vi "Periodic Tasks.vi"(8 "error in":errorcluster) -> ()   [LabVIEW 2015]
doc: "This VI runs in parallel to other tasks. It can contain as many user-defined periodic loops as you need. These can carry out PID or other sorts of timed response."
uses:
  <vilib>/Rock Robotics/WPI/Relay/WPI_RelayValue.ctl
  <vilib>/Rock Robotics/SystemInterfaces/spilib/spi_bus.ctl
  <vilib>/addons/control/pid/pid.llb/PID Structure.ctl
  <vilib>/Rock Robotics/WPI/CAN/TalonSRX/WPI_CANTalonSRX_APIControlMode.ctl
  <vilib>/Rock Robotics/Network Tables/NT Read Number.vi
  Robot Global Data.vi
  <vilib>/Rock Robotics/Network Tables/NT Write Number.vi
  <vilib>/Rock Robotics/WPI/Solenoid/Deprecated/WPI_SolenoidSetBool.vi
  VIs/ConvertVoltageToPercentVbs.vi
  <vilib>/Rock Robotics/Network Tables/NT Write Boolean.vi
  <vilib>/addons/control/pid/pid.llb/PID Control Input Filter (DBL).vi
  <vilib>/addons/control/pid/pid.llb/PID Structure Conversion (DBL).vi
  <vilib>/addons/control/pid/pid.llb/PID (DBL).vi
  <vilib>/Rock Robotics/Network Tables/NT Read Boolean.vi
  <vilib>/Rock Robotics/WPI/Gyro/WPI_GyroXRS450_SPI_Open.vi
  <vilib>/addons/control/pid/NI_PID_pid.lvlib
panel:
  out "Arm Motor Output":dbl
  out "Normalized Value":dbl
  out "Arm Angle":dbl
  in  "Current Limit 2":dbl=5.0
  in  "Driving Power 2":dbl=0.4
  out "current (A)":dbl
  in  "PID Arm Good Range":dbl=3.0
  out "Arm Angle PID 3":dbl
  in  "Arm Angle PID 2":T1={"proportional gain (Kc)"=0.018, "integral time (Ti, min)"=1.25, "derivative time (Td, min)"=1e-05}
  out "Arm PID Output Graph":dbl(graph)
  out "Arm PID Output":dbl
  out "Arm Setpoint PID":dbl
  in  "Arm PID Output Range":cluster{"output high":dbl, "output low":dbl}={"output high"=0.5, "output low"=-0.5} {"output low" format="%.2f"; "output high" format="%.2f"}
  in  "Holding Power":dbl=0.1
  in  "Driving Power":dbl=0.6
  in  "Current Limit":dbl=8.0
  out "Scaled Vision x":dbl
  out "Ball Holder Voltage":dbl
  out "Gyro Resetting":bool
  out "SHOOT":bool
  out "Ball Holder":bool
  in  "D Left":dbl
  in  "D Right":dbl
  out "R Error":dbl(graph)
  out "L Error":dbl(graph)
  in  "I Right":dbl
  in  "I Left":dbl
  out "Shooter Data":T2={"Arm Angle"={"D4"=44.0, "Fender"=69.0, "Low Goal"=-1.0, "Bottom"=-3.0}, "Wheel Speed"={"D4"=4500.0, "Fender"=3600.0, "Low Goal"=3000.0, "Intake"=-11.0}}
  in  "Wheel Speed Setpoints":T3={"D4"=3450.0, "Fender"=3500.0, "Low Goal"=2500.0, "Intake"=-13.0}
  in  "Arm Angle Setpoints":T4={"D4"=38.0, "Fender"=72.0, "Low Goal"=-1.0, "Bottom"=0.0}
  out "Angle":dbl
  in  "Reset Gyro":bool
  out "Speed Closed Loop Plots R":cluster{dbl, "Sensor Velocity":dbl}(graph)
  out "SensorRPM Velocity RPM R":dbl
  out "Target RPM R":dbl
  out "Target RPM L":dbl
  out "SensorRPM Velocity RPM L":dbl
  out "Speed Closed Loop Plots L":cluster{dbl, "Sensor Velocity":dbl}(graph)
  in  "P Right":dbl=0.1
  in  "F Right":dbl=0.02417
  in  "P Left":dbl=0.11
  in  "F Left":dbl=0.025837
  out "Vision X Dashboard":dbl
  out "Vision Y Dashboard":dbl
  out "Average Distance":dbl
  # "Sensor Stuff"
  # "Random Stuff"
  # "Vision Stuff"
  # "Shooter Data"
  # "Arm Angle Control"
  # "-3"
  # "OLD F\n3300"
  # "Shooter Wheel Control"
  # "RIGHT"
  # "50\n50"
  # "Delays to compensate for wheel speed.\n\n1: Wait for wheels to spin up before piston fires\n2: Keep wheels spun up after piston fires"
  # "LEFT"
  # ".45\n.37\n\n.15\n.025"
  # "Arm Angle"
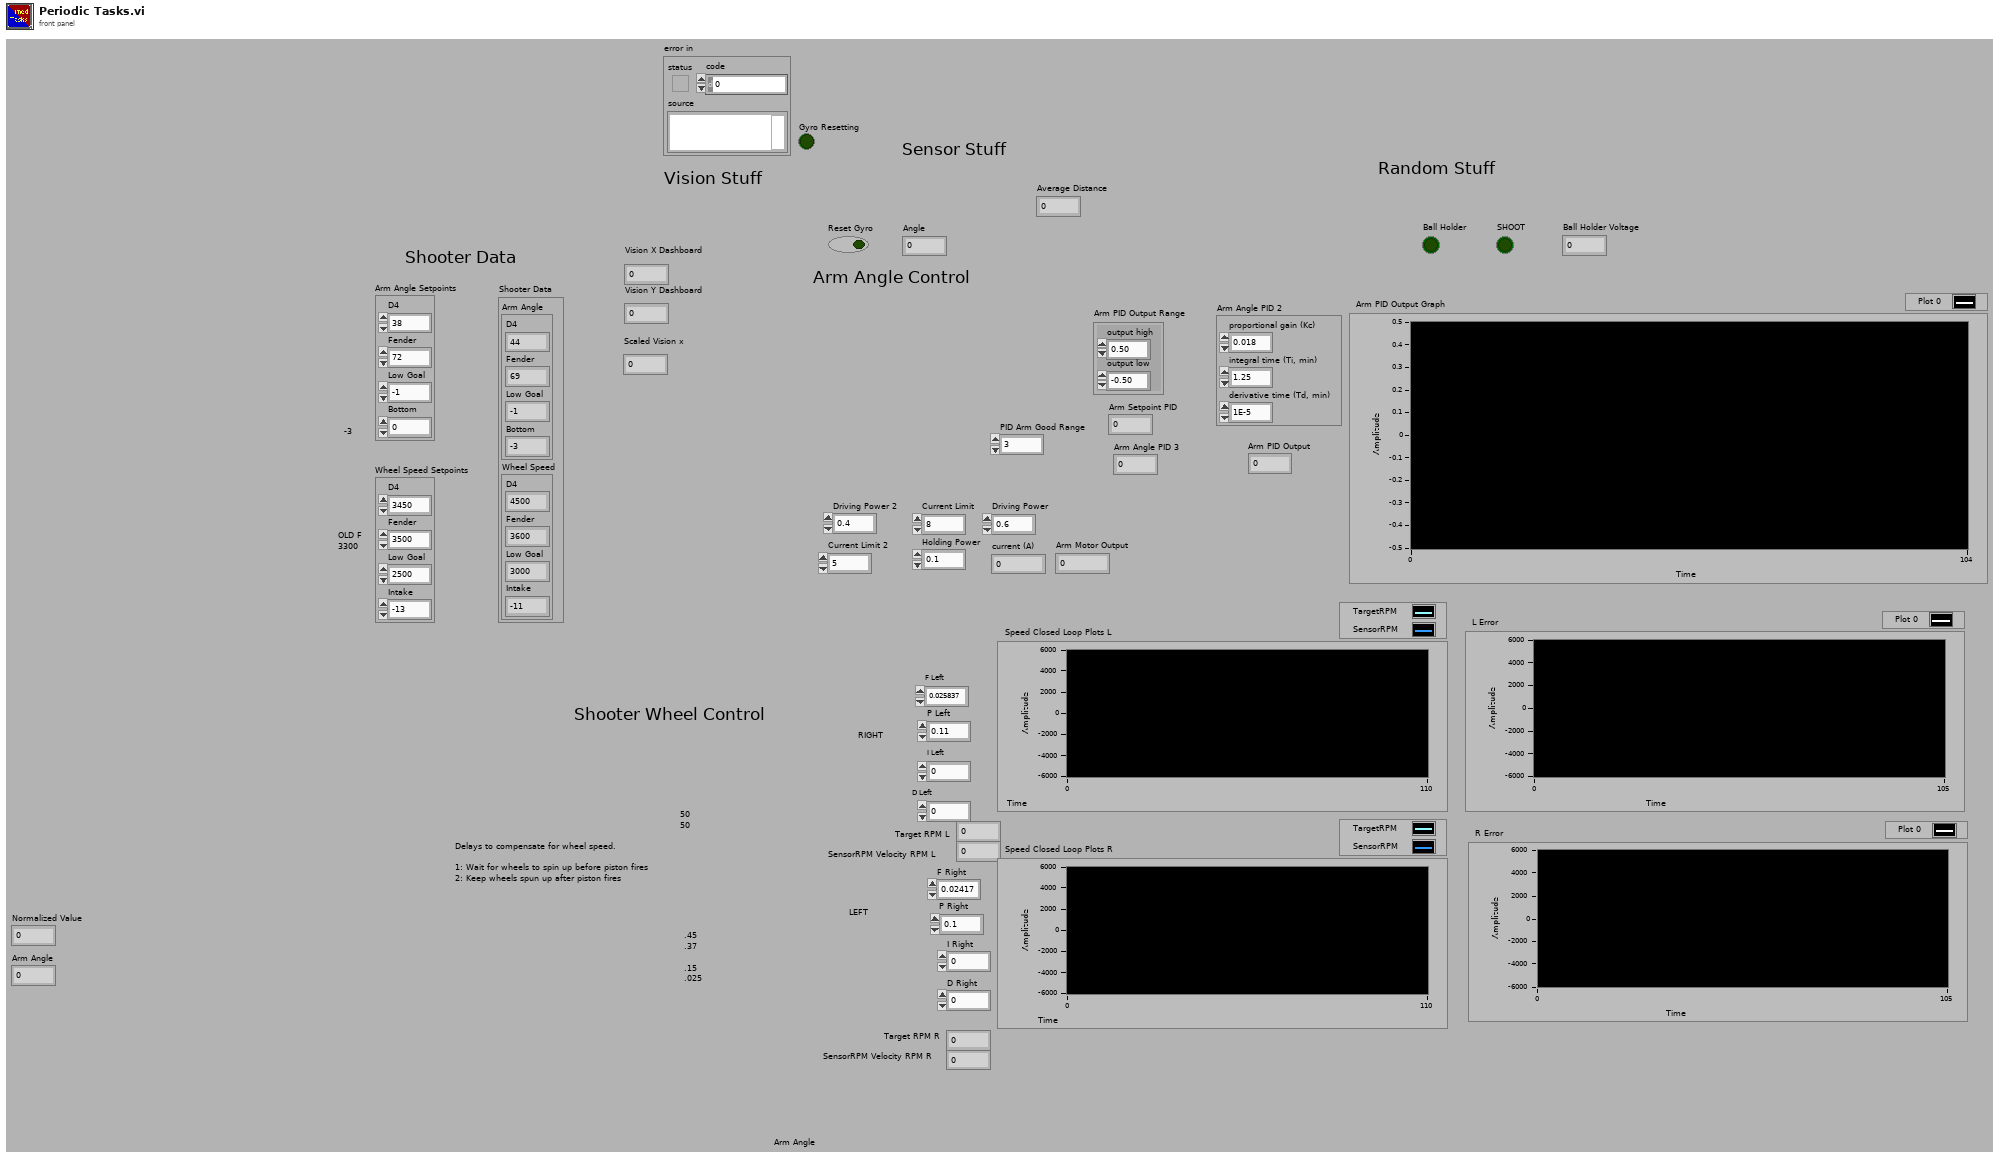
[diagram p1: front panel]
types:
  T1 = cluster{"proportional gain (Kc)":dbl, "integral time (Ti, min)":dbl, "derivative time (Td, min)":dbl}
  T2 = cluster{"Arm Angle":cluster{"D4":dbl, "Fender":dbl, "Low Goal":dbl, "Bottom":dbl}, "Wheel Speed":cluster{"D4":dbl, "Fender":dbl, "Low Goal":dbl, "Intake":dbl}}
  T3 = cluster{"D4":dbl, "Fender":dbl, "Low Goal":dbl, "Intake":dbl}
  T4 = cluster{"D4":dbl, "Fender":dbl, "Low Goal":dbl, "Bottom":dbl}
  T5 = typedef "WPI_PotentiometerDevRef.ctl" = cluster{"DevStatus":errorcluster, "Analog Channel":T6, "Invert Output":bool}
  T6 = typedef "FPGA_AIChannel.ctl" = enum8{"AI 0", "AI 1", "AI 2", "AI 3", "AI MXP 0", "AI MXP 1", "AI MXP 2", "AI MXP 3", "Invalid"}
  T7 = typedef "NI_PID_pid.lvlib/PID Structure.ctl" = u16
  T8 = typedef "WPI_MotorControlDeviceRef.ctl" = cluster{"DeviceStatus":errorcluster, "Type":T9, "PWM":cluster{"PWM Channel":T10, "DeadBand":T11}, "CAN":cluster{"Device Number":u8, "Control Mode":T12, "Semaphore":T13, "Max Vout":dbl, "TalonSRX Control Mode":T14}, "Invert":bool}
  T9 = typedef "WPI_MotorControlType.ctl" = enum16{"PWM", "CAN", "CANTalonSRX"}
  T10 = typedef "FPGA_DIOPWMChannel.ctl" = enum8{"PWM 0", "PWM 1", "PWM 2", "PWM 3", "PWM 4", "PWM 5", "PWM 6", "PWM 7", "PWM 8", "PWM 9", "PWM MXP 0", "PWM MXP 1", "PWM MXP 2", "PWM MXP 3", "PWM MXP 4", "PWM MXP 5", "PWM MXP 6", "PWM MXP 7", "PWM MXP 8", "PWM MXP 9", "Invalid"}
  T11 = typedef "WPI_PWMDeadband.ctl" = cluster{"Name":string, "maxPositivePwm":i32, "minPositivePwm":i32, "centerPwm":i32, "maxNegativePwm":i32, "minNegativePwm":i32, "angularRange":u16}
  T12 = typedef "WPI_CANJaguar_ControlMode.ctl" = enum8{"Percent VBus", "Current", "Speed", "Position", "Voltage"}
  T13 = typedef "Semaphore RefNum" = refnum<k1>
  T14 = typedef "WPI_CANTalonSRX_APIControlMode.ctl" = enum8{"Percent VBus", "Speed", "Position", "Slave", "Unchanged / Invalid", "Voltage Compensation", "Current", "Motion Profile"}
  T15 = typedef "WPI_EncoderDevRef.ctl" = cluster{"DevStatus":errorcluster, "EncoderIndex":T16, "CounterIndex":T17, "DistancePerCount":dbl, "Decoding Type":T18}
  T16 = typedef "FPGA_EncoderIdx.ctl" = enum8{"Enc 0", "Enc 1", "Enc 2", "Enc 3", "Enc 4", "Enc 5", "Enc 6", "Enc 7", "Invalid"}
  T17 = typedef "FPGA_CounterCtrSystemIndex.ctl" = enum8{"Ctr 0", "Ctr 1", "Ctr 2", "Ctr 3", "Ctr 4", "Ctr 5", "Ctr 6", "Ctr 7", "Invalid"}
  T18 = typedef "WPI_EncoderType.ctl" = enum16{"1x", "2x", "4x"}
  T19 = typedef "WPI_GyroDevRef.ctl" = cluster{"DevStatus":errorcluster, "Analog Channel":T6, "Offset":dbl, "Gain (VoltsPerDegree/Second)":dbl, "Gyro Type":enum16{"Analog", "XRS450"}, "Handle":i32, "SPI Bus":T20, "Device Found":bool, "Sample Rate":dbl, "Calibrate On Open":bool}
  T20 = typedef "spi_bus.ctl" = enum16{"SPI On-Board, CS0", "SPI On-Board, CS1", "SPI On-Board, CS2", "SPI On-Board, CS3", "SPI MXP", "Invalid"}
  T21 = typedef "WPI_RelayValue.ctl" = enum16{"Off", "On", "Forward", "Reverse"}
  T22 = typedef "WPI_SolenoidDevRef.ctl" = cluster{"DevStatus":errorcluster, "Pneumatics Control Module":u8, "Forward Solenoid Channel":T23, "Reverse Solenoid Channel":T23}
  T23 = typedef "WPI_SolenoidChannel.ctl" = enum8{"Solenoid 0", "Solenoid 1", "Solenoid 2", "Solenoid 3", "Solenoid 4", "Solenoid 5", "Solenoid 6", "Solenoid 7", "Invalid"}
  T24 = typedef "WPI_RelayDevRef.ctl" = cluster{"DevStatus":errorcluster, "Relay Channel":T25, "Relay Direction":T26}
  T25 = typedef "FPGA_DIORelayChannel.ctl" = enum8{"Relay 0", "Relay 1", "Relay 2", "Relay 3", "Invalid"}
  T26 = typedef "WPI_RelayDirection.ctl" = enum16{"Both directions", "Forward only", "Reverse only"}
  T27 = typedef "WPI_CANTalonSRX_GlobalStatus.ctl" = cluster{"Applied Throttle":dbl, "Module Enabled":bool, "CAN Error":errorcluster, "Closed Loop Error":dbl, "Forward Limit Switch Closed":bool, "Reverse Limit Switch Closed":bool, "Sensor Position":dbl, "Sensor Velocity":dbl, "Current":dbl, "Sticky Fault - Over Temp":bool, "Sticky Fault - Under Voltage":bool, "Sticky Fault - Forward Limit":bool, "Sticky Fault - Reverse Limit":bool, "Sticky Fault - Forward Soft Limit":bool, "Sticky Fault - Reverse Soft Limit":bool, "Brake is Enabled":bool, "Encoder Position":dbl, "Encoder Velocity":dbl, "Encoder Index Count":dbl, "Encoder A Pin State":bool, "Encoder B Pin State":bool, "Encoder Index Pin State":bool, "Analog In":dbl, "Analog In Velocity":dbl, "Temperature (C)":dbl, "Battery Voltage":dbl, "Control 5 Is Supported":bool, "Current Profile Slot Select":dbl, "Pos Div 8":bool, "Vel Div 4":bool, "Pulse Width Position":i32, "Pulse Width Velocity":i32, "Pulse Width Rise To Rise (us)":i32, "Pulse Width Rise To Fall (us)":i32, "Mot Prof Active Is Under Run":bool, "Mot Prof Active Has Under Run":bool, "Mot Prof Active Is Last":bool, "Mot Prof Active Velocity Only":bool, "Mot Prof Active Is Valid":bool, "Mot Prof Buffer Is Full":bool, "Mot Prof Active Profile Slot Select":i32, "Mot Prof NextID":i32, "Mot Prof Count":i32, "Mot Prof Active Velocity":dbl, "Mot Prof Active Position":dbl, "Mot Prof Output Enable":i32}
  T28 = cluster{"Shooter Setpoint Speed (RPM)":dbl, "Sensor Velocity":dbl}
  T29 = typedef "WPI_AnalogChannelDevRef.ctl" = cluster{"DevStatus":errorcluster, "Analog Channel":T6}
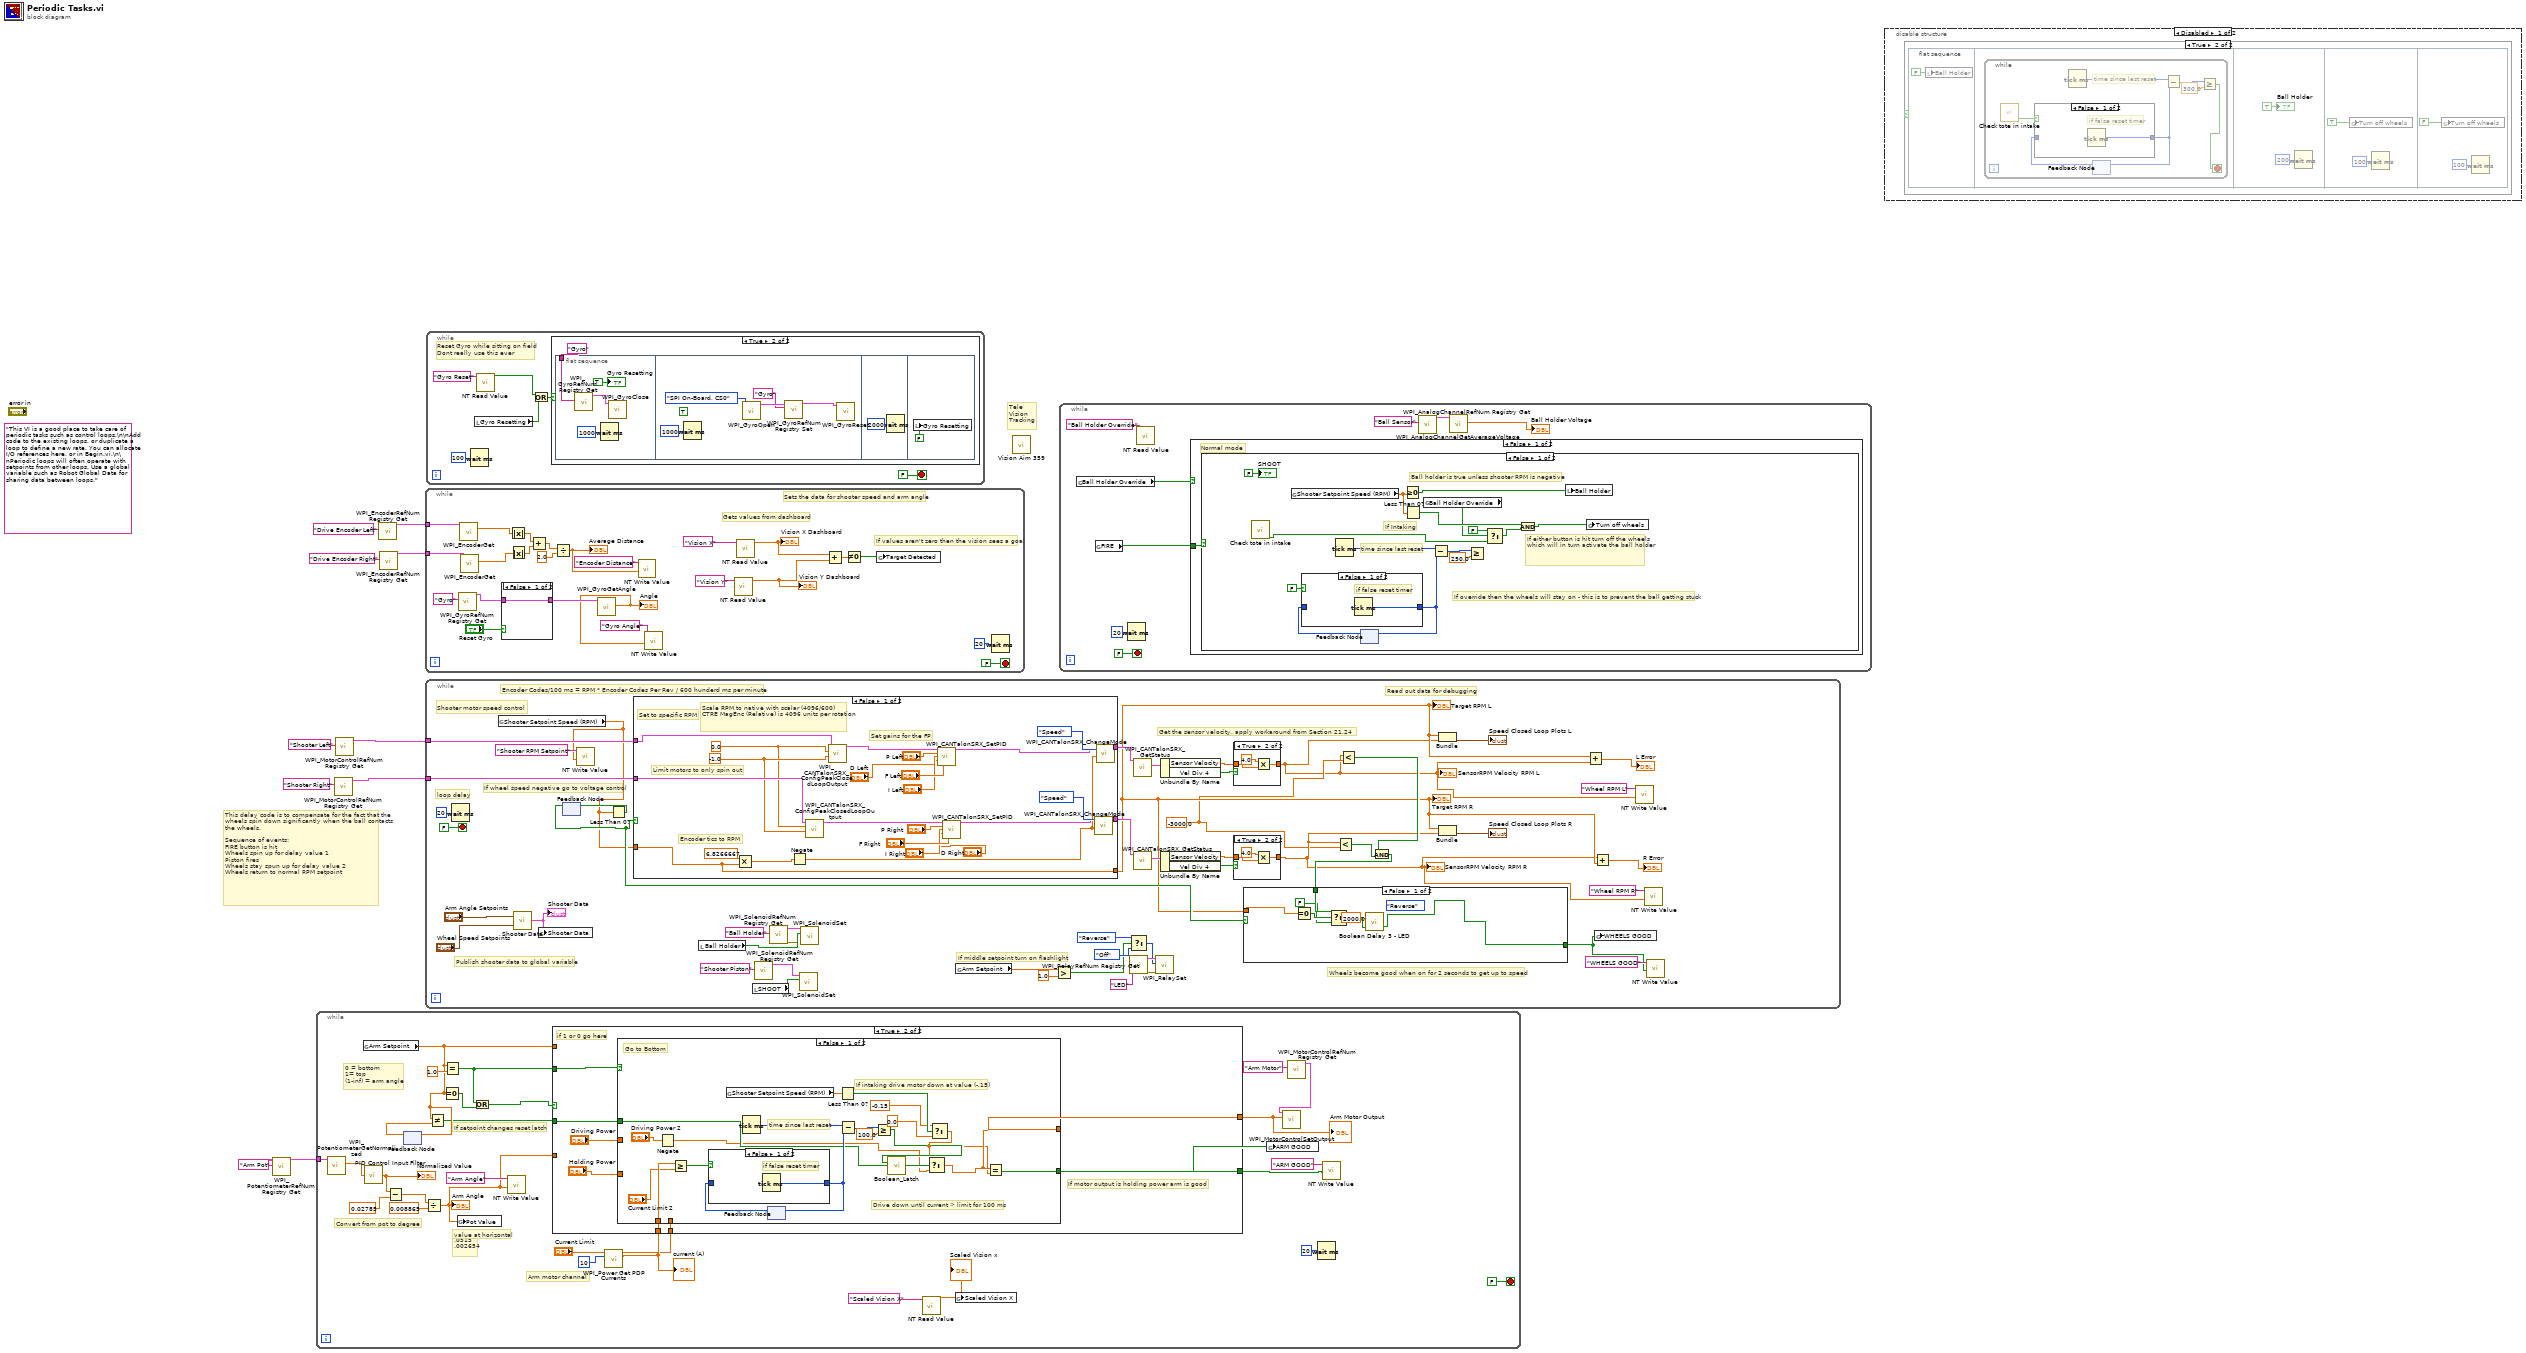
[diagram p0: block diagram]
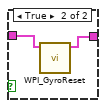
[diagram p2: hidden frame]
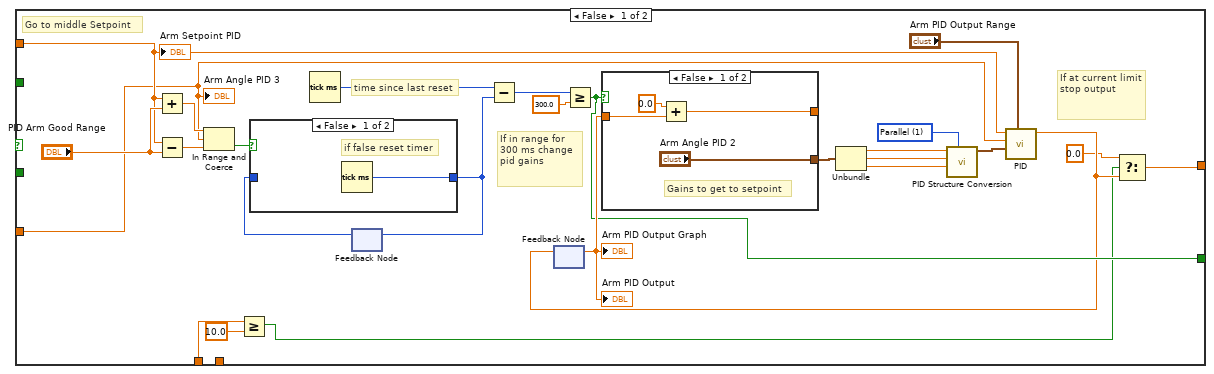
[diagram p6: hidden frame]
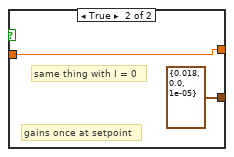
[diagram p8: hidden frame]
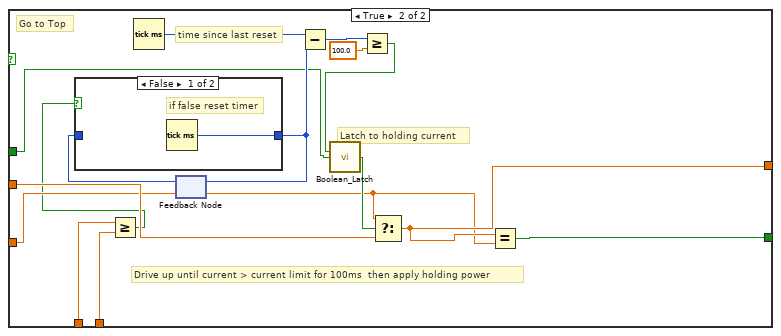
[diagram p10: hidden frame]
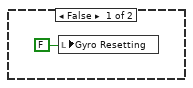
[diagram p12: hidden frame]
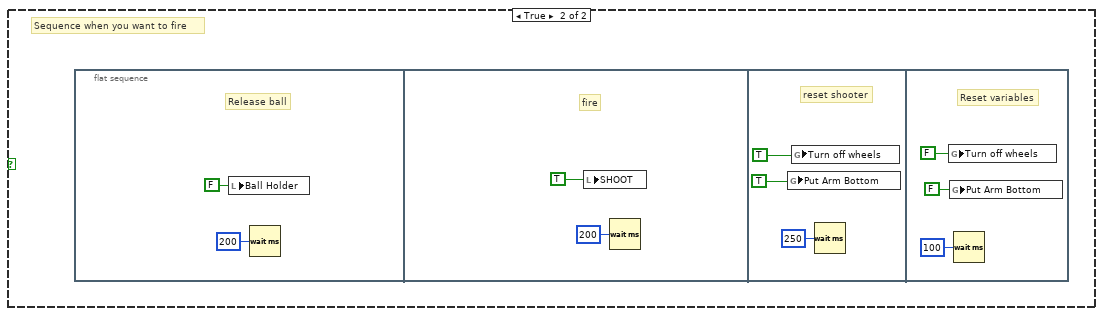
[diagram p14: hidden frame]
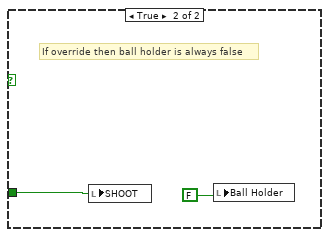
[diagram p15: hidden frame]
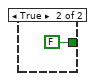
[diagram p16: hidden frame]
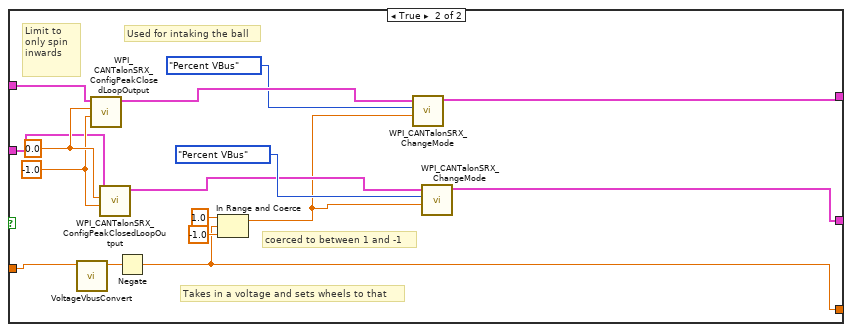
[diagram p19: hidden frame]
diagram:
  (unwired) "This VI is a good place to take care of periodic tasks such as control loops.\n\nAdd code to the existing loops, or duplicate a loop to define a new rate. You can allocate I/O references here, or in Begin.vi.\n\nPeriodic loops will often operate with setpoints from other loops. Use a global variable such as Robot Global Data for sharing data between loops."
  # "Tele \nVision\nTracking"
  # "This delay code is to compensate for the fact that the wheels spin down significantly when the ball contacts the wheels.\n\nSequence of events:\nFIRE button is hit\nWheels spin up for delay value 1\nPiston fires\nWheels stay spun up for delay value 2\nWheels return to normal RPM setpoint"
  n1 = call <vilib>:"WPI_PotentiometerRefNum Registry Get.vi"("refnum name"="Arm Pot") -> ("PotDevRef"=w1:T5)  [unwired: 9 in, 1 out]
  n2 = while {
    tunnel: w1 -> [w17]
    stop <- FALSE stop-if-true
    # "If setpoint changes reset latch"
    # "0 = bottom\n1= top \n(1-inf) = arm angle"
    # "Convert from pot to degree"
    # "value at horizontal"
    # "old\n.0515\n.002654"
    # "Arm motor channel"
    n3 = call <vilib>:"WPI_PotentiometerGetNormalized.vi"("PotDevRef"=w17) -> ("Normalized Value"=w20:dbl)  [unwired: 8 in, 2 out]
    n4 = global read "Robot Global Data.vi" "Arm Setpoint"() -> (w13:dbl)
    n5 = call-poly <vilib>:"PID Control Input Filter.vi"("input"=w20) -> ("output"=w19:dbl)  [unwired: 4 in]
    "Normalized Value" <- w19
    n6 = Subtract(x=w19, y=0.02785) -> (x-y=w23:dbl)
    n7 = feedback-in #1(w13) -> ()
    n8 = feedback #1() -> (w25:dbl)  [unwired: 1 in]
    n9 = Divide(x=w23, y=0.008865) -> (x/y=w18:dbl)
    "Arm Angle" <- w18
    n10 = Not Equal?(x=w13, y=w25) -> (x != y?=w12:bool)
    n11 = Equal To 0?(x=w13) -> (x = 0?=w36:bool)
    n12 = Equal?(x=w13, y=1.0) -> (x = y?=w35:bool)
    n13 = global write "Robot Global Data.vi" "Pot Value"(w18) -> ()
    n14 = Or(x=w35, y=w36) -> (x .or. y?=w11:bool)
    n15 = call-poly <vilib>:"NT Write Value.vi"("Numeric"=w18, "Name"="Arm Angle") -> ()  [unwired: 9 in, 1 out]
    n16 = call <vilib>:"WPI_Power Get PDP Currents.vi"("PDP Channel"=10) -> ("current (A)"=w33:dbl)  [unwired: 12 in, 2 out]
    "current (A)" <- w33
    n17 = case shown="True" w11 {
      tunnel: w35 -> [_ w79]
      tunnel: w33 -> [w43 w78]
      tunnel: "Current Limit" -> [_ w77]
      tunnel: [w45 w74] -> w30
      tunnel: w13 -> [w46 _]
      tunnel: [w41 w73] -> w14
      tunnel: w12 -> [_ w72]
      tunnel: w18 -> [w44 _]
      frame False {
        w50 = T7 1 items=["Academic (Standard)", "Parallel", "Series"] ("PID structure")
        # "If in range for 300 ms change pid gains"
        # "If at current limit stop output"
        # "time since last reset"
        # "Go to middle Setpoint"
        n18 = Add(x=w46, y="PID Arm Good Range") -> (x+y=w48:dbl)
        n19 = Subtract(x=w46, y="PID Arm Good Range") -> (x-y=w49:dbl)
        n20 = In Range and Coerce(upper limit=w48, x=w44, lower limit=w49) -> (In Range?=w62:bool)  [unwired: 1 out]
        n21 = Greater Or Equal?(x=w43, y=10.0) -> (x >= y?=w38:bool)
        n22 = Tick Count (ms)() -> (millisecond timer value=w57:u32)
        n23 = feedback #2() -> (w60:u32)  [unwired: 1 in]
        n24 = case shown="False" w62 {
          tunnel: [w64 w65] -> w58
          tunnel: w60 -> [_ w65]
          frame False {
            # "if false reset timer"
            n25 = Tick Count (ms)() -> (millisecond timer value=w64:u32)
          }
          frame True {
            # "if true don't reset timer"
          }
        }
        n26 = feedback-in #2(w58) -> ()
        n27 = Subtract(x=w57, y=w58) -> (x-y=w59:u32)
        n28 = feedback #3() -> (w56:dbl)  [unwired: 1 in]
        "Arm PID Output" <- w56
        "Arm PID Output Graph" <- w56
        n29 = Greater Or Equal?(x=w59, y=300.0 ("Delay (ms)")) -> (x >= y?=w45:bool)
        n30 = case shown="False" w45 {
          tunnel: ["Arm Angle PID 2" T1 {"proportional gain (Kc)"=0.018, "integral time (Ti, min)"=0.0, "derivative time (Td, min)"=1e-05} ("cluster")] -> w47
          tunnel: [w66 w70] -> _
          tunnel: w56 -> [w68 w70]
          frame False {
            # "Gains to get to setpoint"
            n31 = Add(x=0.0, y=w68) -> (x+y=w66:dbl)
          }
          frame True {
            # "same thing with I = 0"
            # "gains once at setpoint"
          }
        }
        n32 = Unbundle(w47) -> ("proportional gain (Kc)"=w55:dbl, "integral time (Ti, min)"=w54:dbl, "derivative time (Td, min)"=w53:dbl)
        n33 = call-poly <vilib>:"PID Structure Conversion.vi"("PID structure"=w50, "derivative"=w53, "integral"=w54, "proportional"=w55) -> ("PID gains"=w52:T1)  [unwired: 7 in]
        n34 = call-poly <vilib>:"PID.vi"("output range"="Arm PID Output Range", "PID gains"=w52, "process variable"=w44, "setpoint"=w46) -> ("output"=w40:dbl)  [unwired: 6 in, 1 out]
        n35 = feedback-in #3(w40) -> ()
        n36 = Select(t=0.0, s=w38, f=w40) -> (s? t:f=w41:dbl)
        "Arm Setpoint PID" <- w46
        "Arm Angle PID 3" <- w44
      }
      frame True {
        # "If motor output is holding power arm is good"
        # "if 1 or 0 go here"
        n37 = case shown="False" w79 {
          tunnel: w78 -> [w99 w116]
          tunnel: w77 -> [_ w115]
          tunnel: "Holding Power" -> [_ w110]
          tunnel: "Driving Power" -> [_ w111]
          tunnel: [w98 w114] -> w74
          tunnel: [w96 w112] -> w73
          tunnel: w72 -> [w88 w102]
          frame False {
            # "If intaking drive motor down at value (-.15)"
            # "Drive down until current > limit for 100 ms"
            # "time since last reset"
            # "Go to Bottom"
            n38 = Negate(x="Driving Power 2") -> (-x=w87:dbl)
            n39 = Greater Or Equal?(x=w99, y="Current Limit 2") -> (x >= y?=w90:bool)
            n40 = global read "Robot Global Data.vi" "Shooter Setpoint Speed (RPM)"() -> (w82:dbl)
            n41 = Tick Count (ms)() -> (millisecond timer value=w95:u32)
            n42 = feedback #4() -> (w91:u32)  [unwired: 1 in]
            n43 = case shown="False" w90 {
              tunnel: [w100 w101] -> w94
              tunnel: w91 -> [_ w101]
              frame False {
                # "if false reset timer"
                n44 = Tick Count (ms)() -> (millisecond timer value=w100:u32)
              }
              frame True {
                # "if true don't reset timer"
              }
            }
            n45 = feedback-in #4(w94) -> ()
            n46 = Less Than 0?(x=w82) -> (x < 0?=w81:bool)
            n47 = Subtract(x=w95, y=w94) -> (x-y=w93:u32)
            n48 = Greater Or Equal?(x=w93, y=100.0 ("Delay (ms)")) -> (x >= y?=w89:bool)
            n49 = call "Boolean_Latch.vi"("Latch Control"=w89, "Reset"=w88) -> ("Latched?"=w97:bool)  [unwired: 13 in]
            n50 = Select(t=-0.15, s=w81, f=0.0) -> (s? t:f=w83:dbl)
            n51 = Select(t=w83, s=w97, f=w87) -> (s? t:f=w96:dbl)
            n52 = Equal?(x=w96, y=w83) -> (x = y?=w98:bool)
          }
          frame True {
            # "Latch to holding current"
            # "Drive up until current > current limit for 100ms  then apply holding power"
            # "time since last reset"
            # "Go to Top"
            n53 = Greater Or Equal?(x=w116, y=w115) -> (x >= y?=w103:bool)
            n54 = Tick Count (ms)() -> (millisecond timer value=w109:u32)
            n55 = feedback #5() -> (w105:u32)  [unwired: 1 in]
            n56 = case shown="False" w103 {
              tunnel: [w117 w118] -> w108
              tunnel: w105 -> [_ w118]
              frame False {
                # "if false reset timer"
                n57 = Tick Count (ms)() -> (millisecond timer value=w117:u32)
              }
              frame True {
                # "if true don't reset timer"
              }
            }
            n58 = feedback-in #5(w108) -> ()
            n59 = Subtract(x=w109, y=w108) -> (x-y=w107:u32)
            n60 = Greater Or Equal?(x=w107, y=100.0 ("Delay (ms)")) -> (x >= y?=w104:bool)
            n61 = call "Boolean_Latch.vi"("Latch Control"=w104, "Reset"=w102) -> ("Latched?"=w113:bool)  [unwired: 13 in]
            n62 = Select(t=w110, s=w113, f=w111) -> (s? t:f=w112:dbl)
            n63 = Equal?(x=w112, y=w110) -> (x = y?=w114:bool)
          }
        }
      }
    }
    "Arm Motor Output" <- w14
    n64 = call-poly <vilib>:"NT Read Value.vi"("Name"="Scaled Vision X") -> ("Numeric"=w15:dbl)  [unwired: 9 in, 1 out]
    "Scaled Vision x" <- w15
    n65 = global write "Robot Global Data.vi" "Scaled Vision X"(w15) -> ()
    n66 = global write "Robot Global Data.vi" "ARM GOOD"(w30) -> ()
    n67 = call <vilib>:"WPI_MotorControlRefNum Registry Get.vi"("refnum name"="Arm Motor") -> ("MotorControlDevRef"=w26:T8)  [unwired: 9 in, 1 out]
    n68 = call <vilib>:"WPI_MotorControlSetOutput.vi"("Output"=w14, "MotorControlDevRef"=w26) -> ()  [unwired: 7 in, 3 out]
    n69 = Wait (ms)(milliseconds to wait=u32 20) -> ()  [unwired: 1 out]
    n70 = call-poly <vilib>:"NT Write Value.vi"("Boolean"=w30, "Name"="ARM GOOD") -> ()  [unwired: 9 in, 1 out]
  }
  n71 = call <vilib>:"WPI_MotorControlRefNum Registry Get.vi"("refnum name"="Shooter Right") -> ("MotorControlDevRef"=w3:T8)  [unwired: 9 in, 1 out]
  n72 = call <vilib>:"WPI_MotorControlRefNum Registry Get.vi"("refnum name"="Shooter Left") -> ("MotorControlDevRef"=w5:T8)  [unwired: 9 in, 1 out]
  n73 = call <vilib>:"WPI_EncoderRefNum Registry Get.vi"("refnum name"="Drive Encoder Left") -> ("EncoderDevRef"=w7:T15)  [unwired: 9 in, 1 out]
  n74 = call <vilib>:"WPI_EncoderRefNum Registry Get.vi"("refnum name"="Drive Encoder Right") -> ("EncoderDevRef"=w8:T15)  [unwired: 9 in, 1 out]
  n75 = while {
    tunnel: w8 -> [w119]
    tunnel: w7 -> [w120]
    stop <- FALSE stop-if-true
    # "Sets the data for shooter speed and arm angle"
    # "If values aren't zero then the vision sees a goal"
    # "Gets values from dashboard"
    n76 = call <vilib>:"WPI_GyroRefNum Registry Get.vi"("refnum name"="Gyro") -> ("GyroDevRef"=w123:T19)  [unwired: 9 in, 1 out]
    n77 = call <vilib>:"WPI_EncoderGet.vi"("EncoderDevRef"=w120) -> ("Distance"=w126:dbl)  [unwired: 5 in, 5 out]
    n78 = call <vilib>:"WPI_EncoderGet.vi"("EncoderDevRef"=w119) -> ("Distance"=w125:dbl)  [unwired: 5 in, 5 out]
    n79 = case shown="False" "Reset Gyro" {
      tunnel: w123 -> [w143 w145]
      tunnel: [w143 w144] -> w132
      frame False {
      }
      frame True {
        n80 = call <vilib>:"WPI_GyroReset.vi"("GyroDevRef"=w145) -> ("GyroDevRef"=w144:T19)  [unwired: 9 in, 1 out]
      }
    }
    n81 = Absolute Value(x=w126) -> (abs(x)=w138:dbl)
    n82 = Absolute Value(x=w125) -> (abs(x)=w139:dbl)
    n83 = Add(x=w138, y=w139) -> (x+y=w137:dbl)
    n84 = Divide(x=w137, y=2.0) -> (x/y=w128:dbl)
    "Average Distance" <- w128
    n85 = call <vilib>:"WPI_GyroGetAngle.vi"("GyroDevRef"=w132) -> ("Angle"=w130:dbl)  [unwired: 6 in, 4 out]
    "Angle" <- w130
    n86 = call-poly <vilib>:"NT Write Value.vi"("Numeric"=w128, "Name"="Encoder Distance") -> ()  [unwired: 9 in, 1 out]
    n87 = call-poly <vilib>:"NT Write Value.vi"("Numeric"=w130, "Name"="Gyro Angle") -> ()  [unwired: 9 in, 1 out]
    n88 = call-poly <vilib>:"NT Read Value.vi"("Name"="Vision Y") -> ("Numeric"=w127:dbl)  [unwired: 9 in, 1 out]
    "Vision Y Dashboard" <- w127
    n89 = call-poly <vilib>:"NT Read Value.vi"("Name"="Vision X") -> ("Numeric"=w124:dbl)  [unwired: 9 in, 1 out]
    "Vision X Dashboard" <- w124
    n90 = Add(x=w124, y=w127) -> (x+y=w141:dbl)
    n91 = Not Equal To 0?(x=w141) -> (x != 0?=w140:bool)
    n92 = global write "Robot Global Data.vi" "Target Detected"(w140) -> ()
    n93 = Wait (ms)(milliseconds to wait=u32 20) -> ()  [unwired: 1 out]
  }
  n94 = while {
    tunnel: w5 -> [w193]
    tunnel: w3 -> [w192]
    stop <- FALSE stop-if-true
    w166 = -3000.0
    # "Read out data for debugging"
    # "Wheels become good when on for 2 seconds to get up to speed"
    # "If middle setpoint turn on flashlight"
    # "Publish shooter data to global variable"
    # "Shooter motor speed control"
    # "If wheel speed negative go to voltage control"
    # "Get the sensor velocity, apply workaround from Section 21.24"
    # "Encoder Codes/100 ms = RPM * Encoder Codes Per Rev / 600 hunderd ms per minute"
    # "loop delay"
    n95 = Wait (ms)(milliseconds to wait=u32 20) -> ()  [unwired: 1 out]
    n96 = global read "Robot Global Data.vi" "Shooter Setpoint Speed (RPM)"() -> (w171:dbl)
    n97 = call "Shooter Data.vi"("Wheel Speed"="Wheel Speed Setpoints", "Arm Angle"="Arm Angle Setpoints") -> ("Shooter Data"=w157:T2)
    "Shooter Data" <- w157
    n98 = global write "Robot Global Data.vi" "Shooter Data"(w157) -> ()
    n99 = feedback #6() -> (w180:bool)  [unwired: 1 in]
    n100 = call-poly <vilib>:"NT Write Value.vi"("Numeric"=w171, "Name"="Shooter RPM Setpoint") -> ()  [unwired: 9 in, 1 out]
    n101 = Less Than 0?(x=w171) -> (x < 0?=w181:bool)
    n102 = feedback-in #6(w181) -> ()
    n103 = case shown="False" w180 {
      tunnel: w171 -> [w220 w241]
      tunnel: w193 -> [w232 w245]
      tunnel: w192 -> [w231 w244]
      tunnel: [w220 w236] -> w169
      tunnel: [w219 w238] -> w183
      tunnel: [w218 w239] -> w182
      frame False {
        w225 = 0.0 ("Forward Peak Output")
        w226 = -1.0 ("Reverse Peak Output")
        # "Set to specific RPM"
        # "Limit motors to only spin out"
        # "Set gains for the FP"
        # "Encoder tics to RPM"
        # "Scale RPM to native with scalar (4096/600)\nCTRE MagEnc (Relative) is 4096 units per rotation"
        n104 = Multiply(x=6.8266667, y=w220) -> (x*y=w217:dbl)
        n105 = Negate(x=w217) -> (-x=w216:dbl)
        n106 = call <vilib>:"WPI_CANTalonSRX_ConfigPeakClosedLoopOutput.vi"("Reverse Peak Output"=w226, "Forward Peak Output"=w225, "CAN Talon SRX Ref"=w231) -> ("CAN Talon SRX Ref"=w223:T8)  [unwired: 7 in, 1 out]
        n107 = call <vilib>:"WPI_CANTalonSRX_ConfigPeakClosedLoopOutput.vi"("Reverse Peak Output"=w226, "Forward Peak Output"=w225, "CAN Talon SRX Ref"=w232) -> ("CAN Talon SRX Ref"=w227:T8)  [unwired: 7 in, 1 out]
        n108 = call <vilib>:"WPI_CANTalonSRX_SetPID.vi"("CAN Talon SRX Ref"=w227, "P"="P Left", "I"="I Left", "D"="D Left", "F"="F Left") -> ("CAN Talon SRX Ref"=w229:T8)  [unwired: 9 in, 1 out]
        n109 = call <vilib>:"WPI_CANTalonSRX_SetPID.vi"("CAN Talon SRX Ref"=w223, "P"="P Right", "I"="I Right", "D"="D Right", "F"="F Right") -> ("CAN Talon SRX Ref"=w222:T8)  [unwired: 9 in, 1 out]
        n110 = call <vilib>:"WPI_CANTalonSRX_ChangeMode.vi"("Output"=w216, "Control Mode"=WPI_CANTalonSRX_APIControlMode."Speed", "CAN Talon SRX Ref"=w222) -> ("CAN Talon SRX Ref"=w219:T8)  [unwired: 7 in, 1 out]
        n111 = call <vilib>:"WPI_CANTalonSRX_ChangeMode.vi"("Output"=w216, "Control Mode"=WPI_CANTalonSRX_APIControlMode."Speed", "CAN Talon SRX Ref"=w229) -> ("CAN Talon SRX Ref"=w218:T8)  [unwired: 7 in, 1 out]
      }
      frame True {
        w247 = 0.0 ("Forward Peak Output")
        w246 = -1.0 ("Reverse Peak Output")
        # "Takes in a voltage and sets wheels to that"
        # "coerced to between 1 and -1"
        # "Limit to only spin inwards"
        # "Used for intaking the ball"
        n112 = call-poly "VoltageVbusConvert.vi"("Voltage"=w241) -> ("Vbus"=w237:dbl)  [unwired: 10 in]
        n113 = call <vilib>:"WPI_CANTalonSRX_ConfigPeakClosedLoopOutput.vi"("Reverse Peak Output"=w246, "Forward Peak Output"=w247, "CAN Talon SRX Ref"=w245) -> ("CAN Talon SRX Ref"=w251:T8)  [unwired: 7 in, 1 out]
        n114 = call <vilib>:"WPI_CANTalonSRX_ConfigPeakClosedLoopOutput.vi"("Reverse Peak Output"=w246, "Forward Peak Output"=w247, "CAN Talon SRX Ref"=w244) -> ("CAN Talon SRX Ref"=w248:T8)  [unwired: 7 in, 1 out]
        n115 = Negate(x=w237) -> (-x=w236:dbl)
        n116 = In Range and Coerce(upper limit=1.0, x=w236, lower limit=-1.0) -> (coerced(x)=w240:dbl)  [unwired: 1 out]
        n117 = call <vilib>:"WPI_CANTalonSRX_ChangeMode.vi"("Output"=w240, "Control Mode"=WPI_CANTalonSRX_APIControlMode."Percent VBus", "CAN Talon SRX Ref"=w251) -> ("CAN Talon SRX Ref"=w239:T8)  [unwired: 7 in, 1 out]
        n118 = call <vilib>:"WPI_CANTalonSRX_ChangeMode.vi"("Output"=w240, "Control Mode"=WPI_CANTalonSRX_APIControlMode."Percent VBus", "CAN Talon SRX Ref"=w248) -> ("CAN Talon SRX Ref"=w238:T8)  [unwired: 7 in, 1 out]
      }
    }
    "Target RPM L" <- w169
    "Target RPM R" <- w169
    n119 = local read "Ball Holder"() -> (w155:bool)
    n120 = local read "SHOOT"() -> (w149:bool)
    n121 = call <vilib>:"WPI_SolenoidRefNum Registry Get.vi"("refnum name"="Shooter Piston") -> ("SolenoidDevRef"=w150:T22)  [unwired: 9 in, 1 out]
    n122 = call <vilib>:"WPI_SolenoidRefNum Registry Get.vi"("refnum name"="Ball Holder") -> ("error out"=w153:errorcluster, "SolenoidDevRef"=w154:T22)  [unwired: 9 in]
    n123 = call-poly <vilib>:"WPI_SolenoidSet.vi"("Value"=w149, "SolenoidDevRef"=w150) -> ()  [unwired: 8 in, 2 out]
    n124 = call-poly <vilib>:"WPI_SolenoidSet.vi"("error in (no error)"=w153, "Value"=w155, "SolenoidDevRef"=w154) -> ()  [unwired: 7 in, 2 out]
    n125 = global read "Robot Global Data.vi" "Arm Setpoint"() -> (w148:dbl)
    n126 = Greater?(x=w148, y=1.0) -> (0:w147:bool)
    n127 = Select(t=WPI_RelayValue."Reverse" ("RelayValue"), s=w147, f=WPI_RelayValue."Off" ("RelayValue")) -> (s? t:f=w159:T21)
    n128 = call <vilib>:"WPI_RelayRefNum Registry Get.vi"("refnum name"="LED") -> ("error out"=w164:errorcluster, "RelayDevRef"=w163:T24)  [unwired: 9 in]
    n129 = call <vilib>:"WPI_CANTalonSRX_GetStatus.vi"("CAN Talon SRX Ref"=w182) -> ("Talon SRX Status"=w188:T27)  [unwired: 8 in, 2 out]
    n130 = call <vilib>:"WPI_CANTalonSRX_GetStatus.vi"("CAN Talon SRX Ref"=w183) -> ("Talon SRX Status"=w187:T27)  [unwired: 8 in, 2 out]
    n131 = call <vilib>:"WPI_RelaySet.vi"("error in (no error)"=w164, "RelayValue"=w159, "RelayDevRef"=w163) -> ()  [unwired: 7 in, 2 out]
    n132 = Unbundle By Name(w188) -> ("Sensor Velocity"=w191:dbl, "Vel Div 4"=w190:bool)
    n133 = Unbundle By Name(w187) -> ("Sensor Velocity"=w184:dbl, "Vel Div 4"=w185:bool)
    n134 = case shown="True" w190 {
      tunnel: [w208 w210] -> w165
      tunnel: w191 -> [w208 w209]
      frame False {
      }
      frame True {
        n135 = Multiply(x=4.0, y=w209) -> (x*y=w210:dbl)
      }
    }
    "SensorRPM Velocity RPM L" <- w165
    n136 = case shown="True" w185 {
      tunnel: [w204 w206] -> w167
      tunnel: w184 -> [w204 w205]
      frame False {
      }
      frame True {
        n137 = Multiply(x=4.0, y=w205) -> (x*y=w206:dbl)
      }
    }
    "SensorRPM Velocity RPM R" <- w167
    n138 = Less?(x=w167, y=w166) -> (x < y?=w176:bool)
    n139 = Less?(x=w165, y=w166) -> (x < y?=w175:bool)
    n140 = And(x=w175, y=w176) -> (x .and. y?=w179:bool)
    n141 = case shown="False" w180 {
      tunnel: w169 -> [w202 _]
      tunnel: w179 -> [w200 _]
      tunnel: [w196 FALSE ("Output")] -> w168
      frame False {
        (unwired) WPI_RelayValue."Reverse" ("RelayValue")
        n142 = Equal To 0?(x=w202) -> (x = 0?=w201:bool)
        n143 = Select(t=FALSE, s=w201, f=w200) -> (s? t:f=w198:bool)
        n144 = call "Boolean Delay 3 - LED.vi"("Input"=w198, "Delay (ms)"=2000.0) -> ("Output"=w196:bool)  [unwired: 1 in]
      }
      frame True {
      }
    }
    n145 = Bundle("Shooter Setpoint Speed (RPM)"=w169, "Sensor Velocity"=w165) -> (→"Speed Closed Loop Plots L":T28)  [unwired: 1 in]
    n146 = Bundle("Shooter Setpoint Speed (RPM)"=w169, "Sensor Velocity"=w167) -> (→"Speed Closed Loop Plots R":T28)  [unwired: 1 in]
    n147 = Add(x=w169, y=w165) -> (x+y=→"L Error":dbl)
    n148 = Add(x=w167, y=w169) -> (x+y=→"R Error":dbl)
    n149 = global write "Robot Global Data.vi" "WHEELS GOOD"(w168) -> ()
    n150 = call-poly <vilib>:"NT Write Value.vi"("Numeric"=w165, "Name"="Wheel RPM L") -> ()  [unwired: 9 in, 1 out]
    n151 = call-poly <vilib>:"NT Write Value.vi"("Numeric"=w167, "Name"="Wheel RPM R") -> ()  [unwired: 9 in, 1 out]
    n152 = call-poly <vilib>:"NT Write Value.vi"("Boolean"=w168, "Name"="WHEELS GOOD") -> ()  [unwired: 9 in, 1 out]
  }
  n153 = while {
    stop <- FALSE stop-if-true
    # "Reset Gyro while sitting on field\nDont really use this ever"
    n154 = Wait (ms)(milliseconds to wait=u32 100) -> ()  [unwired: 1 out]
    n155 = local read "Gyro Resetting"() -> (w252:bool)
    n156 = call-poly <vilib>:"NT Read Value.vi"("Name"="Gyro Reset") -> ("Boolean"=w254:bool)  [unwired: 9 in, 1 out]
    n157 = Or(x=w254, y=w252) -> (x .or. y?=w255:bool)
    n158 = case shown="True" w255 {
      frame False {
        n159 = local write "Gyro Resetting"(FALSE) -> ()
      }
      frame True {
        n160 = flat-sequence {
          tunnel: "Gyro" ("refnum name") -> [w263]
          frame #0 {
            n161 = call <vilib>:"WPI_GyroRefNum Registry Get.vi"("refnum name"=w263) -> ("GyroDevRef"=w262:T19)  [unwired: 9 in, 1 out]
            n162 = Wait (ms)(milliseconds to wait=u32 1000) -> ()  [unwired: 1 out]
            n163 = call <vilib>:"WPI_GyroClose.vi"("GyroDevRef"=w262) -> ()  [unwired: 10 in, 1 out]
            "Gyro Resetting" <- TRUE ("Gyro Resetting")
          }
          frame #1 {
            (unwired) TRUE ("Calibrate On Open")
            n164 = Wait (ms)(milliseconds to wait=u32 1000) -> ()  [unwired: 1 out]
            n165 = call-poly <vilib>:"WPI_GyroOpen.vi"("SPI Bus"=spi_bus."SPI On-Board, CS0") -> ("GyroDevRef"=w268:T19)  [unwired: 9 in, 1 out]
            n166 = call <vilib>:"WPI_GyroRefNum Registry Set.vi"("refnum name"="Gyro", "GyroDevRef"=w268) -> ("GyroDevRef"=w267:T19)  [unwired: 8 in, 1 out]
            n167 = call <vilib>:"WPI_GyroReset.vi"("GyroDevRef"=w267) -> ()  [unwired: 9 in, 2 out]
          }
          frame #2 {
            n168 = Wait (ms)(milliseconds to wait=u32 2000) -> ()  [unwired: 1 out]
          }
          frame #3 {
            n169 = local write "Gyro Resetting"(FALSE) -> ()
          }
        }
      }
    }
  }
  n170 = call "Vision Aim 359.vi"() -> ()  [unwired: 8 in, 4 out]
  n171 = while {
    stop <- FALSE stop-if-true
    n172 = global read "Robot Global Data.vi" "Ball Holder Override"() -> (w275:bool)
    n173 = global read "Robot Global Data.vi" "FIRE"() -> (w277:bool)
    n174 = Wait (ms)(milliseconds to wait=u32 20) -> ()  [unwired: 1 out]
    n175 = call-poly <vilib>:"NT Read Value.vi"("Name"="Ball Holder Override") -> ()  [unwired: 9 in, 2 out]
    n176 = case shown="False" w275 {
      tunnel: w277 -> [w279 w308]
      frame False {
        # "Normal mode"
        n177 = case shown="False" w279 {
          frame False {
            # "If override then the wheels will stay on - this is to prevent the ball getting stuck"
            # "If either button is hit turn off the wheels which will in turn activate the ball holder"
            # "Ball holder is true unless shooter RPM is negative"
            # "time since last reset"
            # "If Intaking"
            n178 = call "Check tote in intake.vi"() -> ("Either"=w282:bool)  [unwired: 8 in, 3 out]
            n179 = global read "Robot Global Data.vi" "Shooter Setpoint Speed (RPM)"() -> (w292:dbl)
            n180 = Tick Count (ms)() -> (millisecond timer value=w290:u32)
            n181 = feedback #7() -> (w286:u32)  [unwired: 1 in]
            n182 = case shown="False" FALSE {
              tunnel: [w295 w296] -> w289
              tunnel: w286 -> [_ w296]
              frame False {
                # "if false reset timer"
                n183 = Tick Count (ms)() -> (millisecond timer value=w295:u32)
              }
              frame True {
                # "if true don't reset timer"
              }
            }
            n184 = feedback-in #7(w289) -> ()
            n185 = Greater Or Equal To 0?(x=w292) -> (x >= 0?=w293:bool)
            n186 = Less Than 0?(x=w292) -> (x < 0?=w291:bool)
            n187 = global read "Robot Global Data.vi" "Ball Holder Override"() -> (w283:bool)
            n188 = Subtract(x=w290, y=w289) -> (x-y=w288:u32)
            n189 = Greater Or Equal?(x=w288, y=250.0 ("Delay (ms)")) -> ()  [unwired: 1 out]
            n190 = Select(t=FALSE, s=w283, f=w282) -> (s? t:f=w280:bool)
            n191 = And(x=w291, y=w280) -> (x .and. y?=w285:bool)
            n192 = local write "Ball Holder"(w293) -> ()
            n193 = global write "Robot Global Data.vi" "Turn off wheels"(w285) -> ()
            "SHOOT" <- FALSE ("SHOOT")
          }
          frame True {
            # "Sequence when you want to fire"
            n194 = flat-sequence {
              frame #0 {
                # "Release ball"
                n195 = local write "Ball Holder"(FALSE ("Ball Holder")) -> ()
                n196 = Wait (ms)(milliseconds to wait=u32 200) -> ()  [unwired: 1 out]
              }
              frame #1 {
                # "fire"
                n197 = local write "SHOOT"(TRUE ("Ball Holder")) -> ()
                n198 = Wait (ms)(milliseconds to wait=u32 200) -> ()  [unwired: 1 out]
              }
              frame #2 {
                # "reset shooter"
                n199 = global write "Robot Global Data.vi" "Put Arm Bottom"(TRUE ("Ball Holder")) -> ()
                n200 = global write "Robot Global Data.vi" "Turn off wheels"(TRUE ("Ball Holder")) -> ()
                n201 = Wait (ms)(milliseconds to wait=u32 250) -> ()  [unwired: 1 out]
              }
              frame #3 {
                # "Reset variables"
                n202 = global write "Robot Global Data.vi" "Turn off wheels"(FALSE ("Ball Holder")) -> ()
                n203 = global write "Robot Global Data.vi" "Put Arm Bottom"(FALSE ("Ball Holder")) -> ()
                n204 = Wait (ms)(milliseconds to wait=u32 100) -> ()  [unwired: 1 out]
              }
            }
          }
        }
      }
      frame True {
        # "If override then ball holder is always false"
        n205 = local write "SHOOT"(w308) -> ()
        n206 = local write "Ball Holder"(FALSE ("Ball Holder")) -> ()
      }
    }
    n207 = call <vilib>:"WPI_AnalogChannelRefNum Registry Get.vi"("refnum name"="Ball Sensor") -> ("AIDeviceRef"=w273:T29)  [unwired: 9 in, 1 out]
    n208 = call <vilib>:"WPI_AnalogChannelGetAverageVoltage.vi"("AIDeviceRef"=w273) -> ("Voltage"=→"Ball Holder Voltage":dbl)  [unwired: 8 in, 2 out]
  }
  n209 = disable-structure shown="Disabled" {
    frame Disabled {
      n210 = case shown="True" {
        selector: _ -> [_ _]
        frame False {
        }
        frame True {
          n211 = flat-sequence {
            frame #0 {
              n212 = local write "Ball Holder"(FALSE ("Ball Holder")) -> ()
            }
            frame #1 {
              n213 = while {
                stop <- w310 stop-if-true
                # "time since last reset"
                n214 = call "Check tote in intake.vi"() -> ("Either"=w312:bool)  [unwired: 8 in, 3 out]
                n215 = Tick Count (ms)() -> (millisecond timer value=w316:u32)
                n216 = feedback #8() -> (w311:u32)  [unwired: 1 in]
                n217 = case shown="False" w312 {
                  tunnel: [w317 w318] -> w315
                  tunnel: w311 -> [_ w318]
                  frame False {
                    # "if false reset timer"
                    n218 = Tick Count (ms)() -> (millisecond timer value=w317:u32)
                  }
                  frame True {
                    # "if true don't reset timer"
                  }
                }
                n219 = feedback-in #8(w315) -> ()
                n220 = Subtract(x=w316, y=w315) -> (x-y=w314:u32)
                n221 = Greater Or Equal?(x=w314, y=300.0 ("Delay (ms)")) -> (x >= y?=w310:bool)
              }
            }
            frame #2 {
              n222 = Wait (ms)(milliseconds to wait=u32 200) -> ()  [unwired: 1 out]
              "Ball Holder" <- TRUE ("Ball Holder")
            }
            frame #3 {
              n223 = global write "Robot Global Data.vi" "Turn off wheels"(TRUE ("Ball Holder Override")) -> ()
              n224 = Wait (ms)(milliseconds to wait=u32 100) -> ()  [unwired: 1 out]
            }
            frame #4 {
              n225 = global write "Robot Global Data.vi" "Turn off wheels"(FALSE ("Ball Holder Override")) -> ()
              n226 = Wait (ms)(milliseconds to wait=u32 100) -> ()  [unwired: 1 out]
            }
          }
        }
      }
    }
    frame Enabled {
    }
  }
